vi "ClosedLoop16_Processing_loop2.vi"(0 "Index of for loop":i32, 1 "element":T1, 2 "Doppler 2D":bool=TRUE, 3 "velocity_profile 3":dbl[][](array[numeric]), 4 "Image Avg":dbl=1.0 min=1.0 max=100.0 step=1.0, 5 "first row":dbl[](array[numeric]), 6 "output cluster":T2, 7 "Power 2D":dbl=0.2 min=0.01 max=0.9 step=0.01, 8 "Num of cross-section per image":i32, 9 "Period":dbl, 11 "ROI":cluster{"ROI_Bot":i32, "ROI_Top":i32}, 13 "Direct Dpp":bool=TRUE, 15 "# Cores":i32=4, 17 "Array":dbl[][](array[numeric]), 19 "Stop Button":bool) -> (14 "Depth profile 2":dbl[][](array[numeric]), 20 "FFT":dbl[](array[numeric]), 21 "velocity_profile shift register":dbl[][](array[numeric]), 22 "Frm#, SmDpp":T3, 23 "Doppler 2D":dbl[][](array[numeric]), 24 "error out 4":errorcluster)   [LabVIEW 2017]
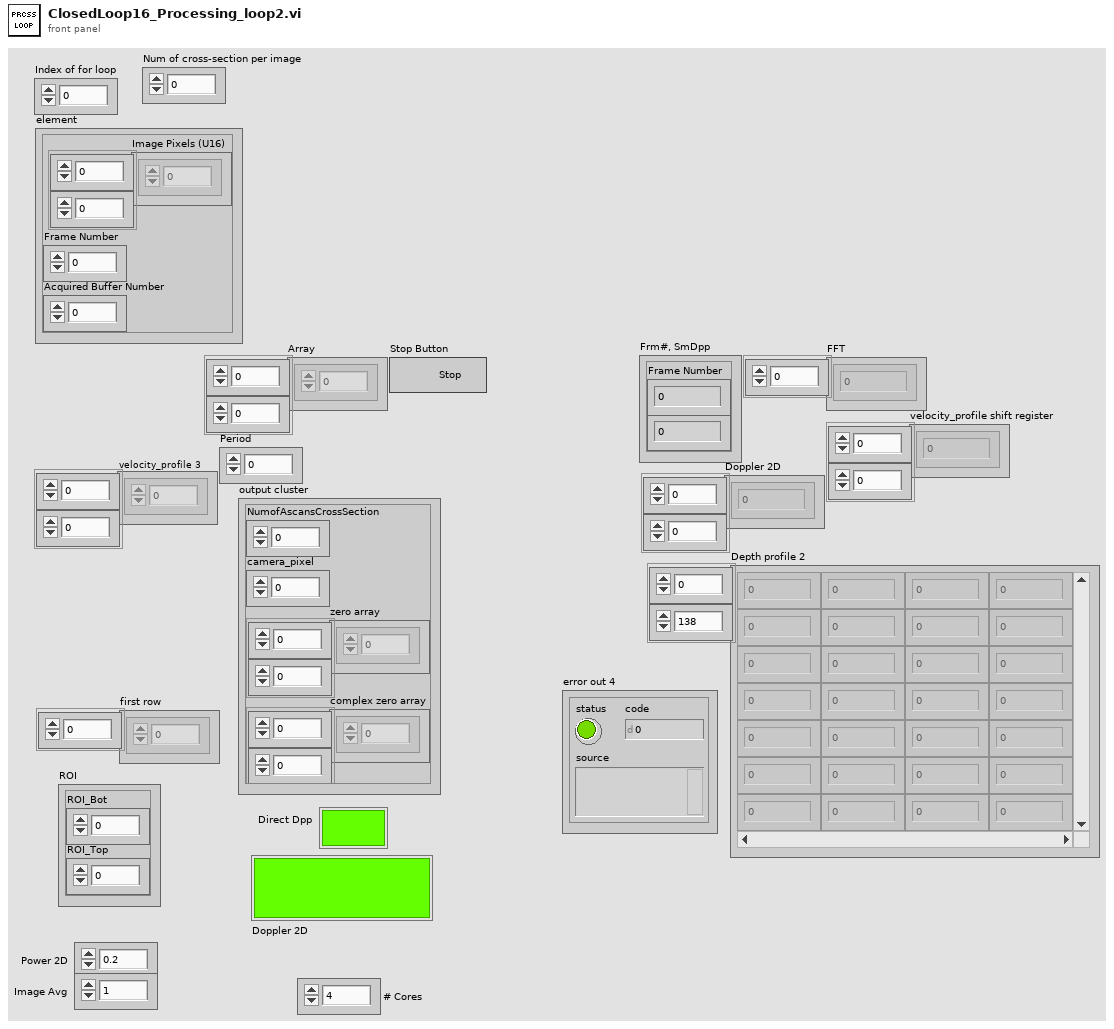
[diagram p1: front panel]
types:
  T1 = cluster{"Image Pixels (U16)":u16[][], "Frame Number":dbl, "Acquired Buffer Number":dbl}
  T2 = cluster{"NumofAscansCrossSection":i32, "camera_pixel":i32, "zero array":dbl[][], "complex zero array":dbl[][]}
  T3 = cluster{"Frame Number":dbl, "Numeric Control":dbl}
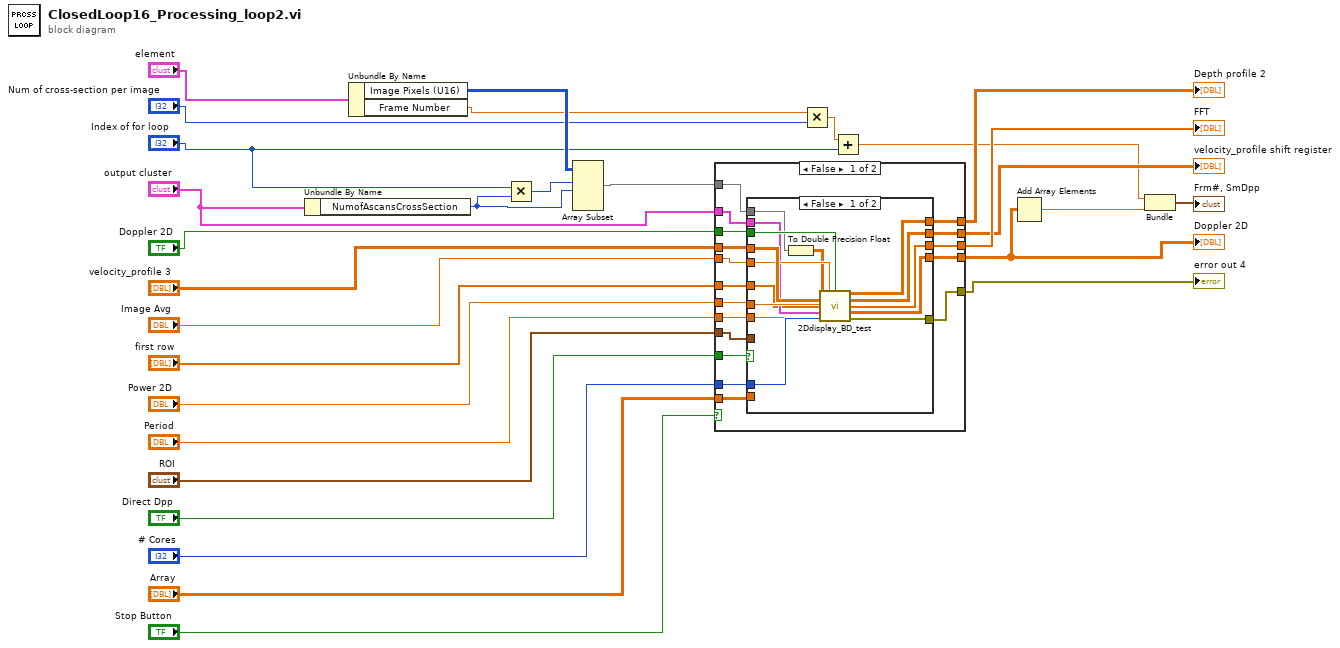
[diagram p0: block diagram]
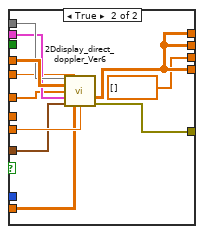
[diagram p2: hidden frame]
diagram:
  n1 = Unbundle By Name("output cluster") -> ("NumofAscansCrossSection"=w3:i32)
  n2 = Unbundle By Name("element") -> ("Image Pixels (U16)"=w27:u16[][], "Frame Number"=w7:dbl)
  n3 = Multiply(x="Index of for loop", y=w3) -> (x*y=w8:i32)
  n4 = Array Subset(array=w27, index (row)=w8, length (row)=w3) -> (w12:u16[][])  [unwired: 2 in]
  n5 = case shown="False" "Stop Button" {
    tunnel: "first row" -> [w46 _]
    tunnel: "output cluster" -> [w41 _]
    tunnel: "velocity_profile 3" -> [w45 w74]
    tunnel: [w44 _] -> w15
    tunnel: [w43 w74] -> w9
    tunnel: "Period" -> [w42 _]
    tunnel: [w40 w73] -> w21
    tunnel: "Doppler 2D" -> [w39 _]
    tunnel: "Image Avg" -> [w38 _]
    tunnel: [w37 _] -> w25
    tunnel: "Power 2D" -> [w36 _]
    tunnel: "Direct Dpp" -> [w35 _]
    tunnel: [w34 _] -> w24
    tunnel: w12 -> [w33 _]
    tunnel: "ROI" -> [w32 _]
    tunnel: "# Cores" -> [w31 _]
    tunnel: "Array" -> [w30 w73]
    frame False {
      n6 = case shown="False" w35 {
        tunnel: w46 -> [w50 w62]
        tunnel: w45 -> [w61 w72]
        tunnel: [w53 w70] -> w44
        tunnel: [w56 w69] -> w43
        tunnel: w42 -> [w47 w71]
        tunnel: w41 -> [w51 w65]
        tunnel: [w54 w69] -> w40
        tunnel: w39 -> [w58 _]
        tunnel: w38 -> [w59 w64]
        tunnel: [w57 w69] -> w37
        tunnel: w36 -> [w60 _]
        tunnel: [w55 dbl[] [] ("Image 2")] -> w34
        tunnel: w33 -> [w49 w66]
        tunnel: w32 -> [_ w67]
        tunnel: w31 -> [w52 _]
        tunnel: w30 -> [_ w63]
        frame False {
          n7 = To Double Precision Float(number=w49) -> (double precision float=w48:dbl[][])
          n8 = call "2Ddisplay_BD_test.vi"("data"=w48, "Image Avg 2D"=w59, "Doppler 2D"=w58, "zero array"=w61, "first row"=w50, "input cluster 3"=w51, "# of Cores"=w52, "Power 2D"=w60, "Period"=w47) -> ("Image"=w57:dbl[][], "buffer out"=w56:dbl[][], "Image 2"=w55:dbl[], "velocity_profile"=w54:dbl[][], "error out"=w53:errorcluster)  [unwired: 2 in]
        }
        frame True {
          n9 = call "2Ddisplay_direct_doppler_Ver6.vi"("Data"=w66, "Image Avg 2D"=w64, "zero array"=w72, "first row"=w62, "input cluster 3"=w65, "ROI"=w67, "VelcityProfile"=w63, "Numeric"=w71) -> ("velocity_profile"=w69:dbl[][], "error out 4"=w70:errorcluster)  [unwired: 5 in, 1 out]
        }
      }
    }
    frame True {
    }
  }
  "Doppler 2D" <- w21
  "FFT" <- w24
  "Depth profile 2" <- w25
  "velocity_profile shift register" <- w9
  "error out 4" <- w15
  n10 = Multiply(x=w7, y="Num of cross-section per image") -> (x*y=w5:dbl)
  n11 = Add(x=w5, y="Index of for loop") -> (x+y=w4:dbl)
  n12 = Add Array Elements(numeric array=w21) -> (sum=w13:dbl)
  n13 = Bundle(w4, "element"=w13) -> (→"Frm#, SmDpp":cluster{dbl, "element":dbl})  [unwired: 1 in]
